vi "USBCAM_FGV.vi"(8 "error in (no error)":errorcluster, 9 "Operation (Read)":enum16{"Write", "Read"}(ring)=enum."Read", 11 "Session In":T1) -> (0 "error out":errorcluster, 3 "Session Out":T1)   [LabVIEW 2020]
uses:
  <vilib>/userDefined/High Color/IMAQdx.ctl
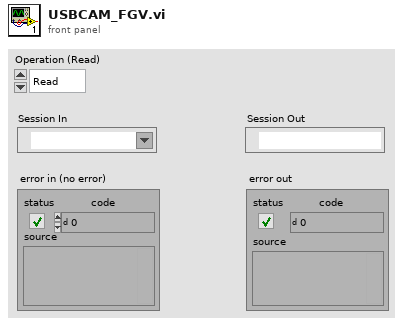
[diagram p1: front panel]
types:
  T1 = typedef "IMAQdx.ctl" = refnum<k21>
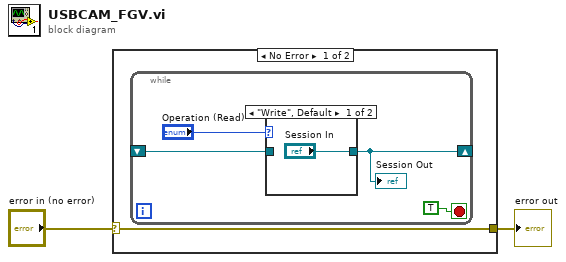
[diagram p0: block diagram]
diagram:
  n1 = case shown="No Error" "error in (no error)" {
    selector: "error in (no error)" -> [w3 w10]
    tunnel: [w3 w10] -> w1
    frame No Error {
      n2 = while {
        shift-right: [w4] -> _
        shift-left: _ -> [w5]
        stop <- TRUE stop-if-true
        n3 = case shown="\"Write\", Default" "Operation (Read)" {
          tunnel: ["Session In" w9] -> w4
          tunnel: w5 -> [_ w9]
          frame "Write", Default {
          }
          frame "Read" {
          }
        }
        "Session Out" <- w4
      }
    }
    frame Error {
    }
  }
  "error out" <- w1
